vi "Set Timestamp Time of Day.vi"(2 "ToD":timestamp, 3 "Time Stamp":timestamp) -> (1 "Time Stamp out":timestamp)   [LabVIEW 2020, in "ARecurrence.lvclass"]
uses:
  ARecurrence.lvclass
  ARecurrence.lvclass/ARecurrence.ctl
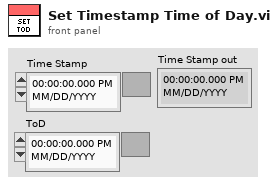
[diagram p1: front panel]
types:
  T1 = typedef "LVDateTimeRec.ctl" = cluster{"fractional second":dbl, "second":i32, "minute":i32, "hour":i32, "day of month":i32, "month":i32, "year":i32, "day of week":i32, "day of year":i32, "DST":i32}
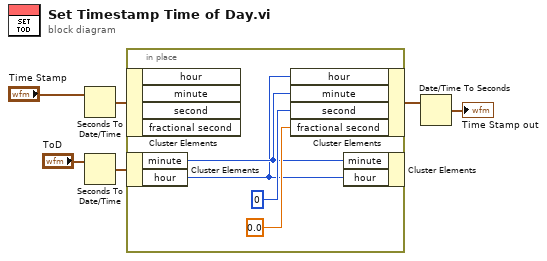
[diagram p0: block diagram]
diagram:
  n1 = Seconds To Date/Time(time stamp (now)="Time Stamp") -> (date time rec=w5:T1)  [unwired: 1 in]
  n2 = Seconds To Date/Time(time stamp (now)="ToD") -> (date time rec=w4:T1)  [unwired: 1 in]
  n3 = in-place {
    n4 = in-place-cluster #1(w5) -> ()  [unwired: 4 out]
    n5 = in-place-cluster #2(w4) -> ("minute"=w8:i32, "hour"=w7:i32)
    n6 = in-place-cluster #1("hour"=w7, "minute"=w8, "second"=0, "fractional second"=0.0) -> (w2:T1)
    n7 = in-place-cluster #2("minute"=w8, "hour"=w7) -> ()  [unwired: 1 out]
  }
  n8 = Date/Time To Seconds(2:w2) -> (0:→"Time Stamp out":timestamp)  [unwired: 1 in]
